vi "Simulation - Tank Level RT.vi"() -> ()   [LabVIEW 2025]
doc: "This example demonstrates a process simulation for a tank level. The process has added noise, valve deadband, lag, and deadtime. A level controller adjusts the inflow to a tank. An on/off valve serves as a drain that you can click on to operate. This s-valve represents a change in the process loading. You also can switch this VI from automatic control to manual control."
uses:
  <vilib>/addons/control/pid/pid.llb/PID Advanced (DBL).vi
  <vilib>/addons/control/pid/NI_PID_pid.lvlib
panel:
  in  "stop":bool
  in  "Tab Control":enum32{"Introduction", "Operation"}(tab)=enum."Operation"
  out "Flow sensor":bool
  in  "HV-101":bool
  out "tank level":dbl(slide)=34.9807513469828 scale=0.0..100.0 scale format="%#.2g"
  out "Valve":bool=TRUE
  in  "LCV-101":dbl(knob)=47.725128287407514 scale=0.0..100.0
  in  "Auto":bool=TRUE
  out "Process Chart":T1(graph)={"initial PV"=34.9807513469828, "SP(%)"=35.294117647058826, "output"=47.725128287407514}
  in  "Setpoint":dbl(slide)=35.294117647058826 scale=0.0..100.0
  in  "PID parameters (LIC 101)":T2={"Kc"=4.0, "Ti (min)"=0.005, "Td (min)"=0.0} {"Td (min)" format="%#.6f"; "Ti (min)" format="%#.4f"; "Kc" format="%#.4f"}
  # "Tank Level Control"
  # "Overview: This example demonstrates a process simulation for a tank level.  The process has added noise, valve deadband, lag, and deadtime.  A level controller adjusts the inflow to a tank.  An on/off valve serves as a drain that you can click on to operate.  This s-valve represents a change in the process loading.  You also can switch this VI from automatic control to manual control.\nInstructions:\n1. Run the VI.\n2. Verify the PID controller in closed-loop to track the setpoint.\n3. Change the setpoint to another value and verify the controller tracking the new setpoint.\n4. Apply a disturbance to the system by switching the valve HV 102 (click on the valve symbol). You will see the controller recovering fro the change.\n5. Change PID gains and see if you can improve its performance without going unstable.\n6. Switch to manual mode and see if you can control the level by changing the Valve LVC 101.\n7. Click Stop to stop the VI."
  # "ISA Symbology: The diagram uses the ISA Symbology used for control"
  # "Loop 101"
  # "Level Controller at the control room"
  # "Level Transmitter on the field"
  # "Level Control Valve on the field"
  # "Hand Control Valve on the field"
  # "HV"
  # "102"
  # "LCV"
  # "101"
  # "LIC"
  # "101"
  # "LT"
  # "101"
  # "Slow Leak"
  # "Click to operate"
  # "HV"
  # "102"
  # "LCV"
  # "101"
  # "LIC"
  # "101"
  # "LT"
  # "101"
  # "Manual"
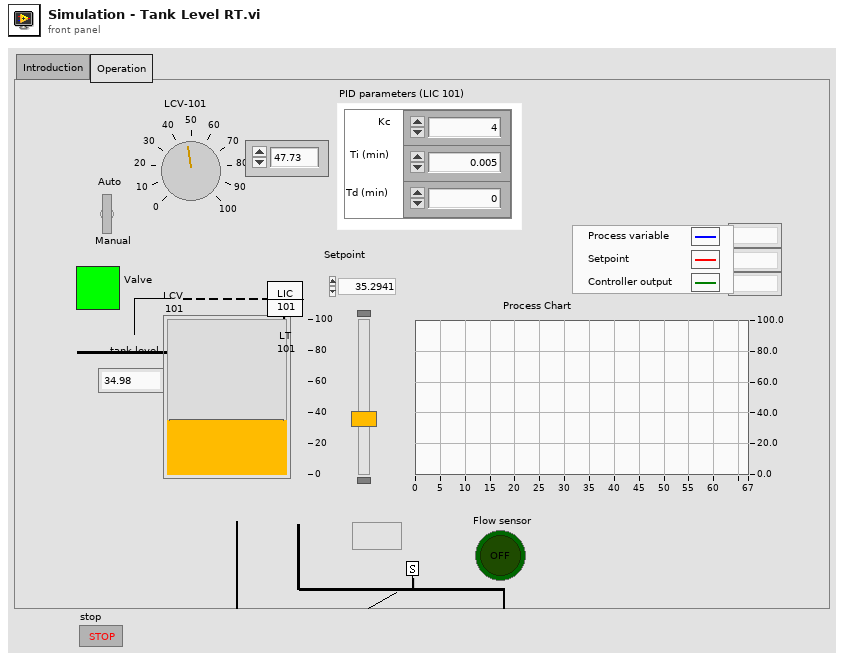
[diagram p1: front panel]
types:
  T1 = cluster{"initial PV":dbl, "SP(%)":dbl, "output":dbl}
  T2 = cluster{"Kc":dbl, "Ti (min)":dbl, "Td (min)":dbl}
  T3 = cluster{"static gain":dbl, "lag (s)":dbl, "deadtime (s)":dbl, "load":dbl, "deadband":dbl, "sensor noise":dbl, "initial PV":dbl, "plant noise":dbl}
  T4 = cluster{"Plant Output":dbl, "Setpoint":dbl, "output":dbl}
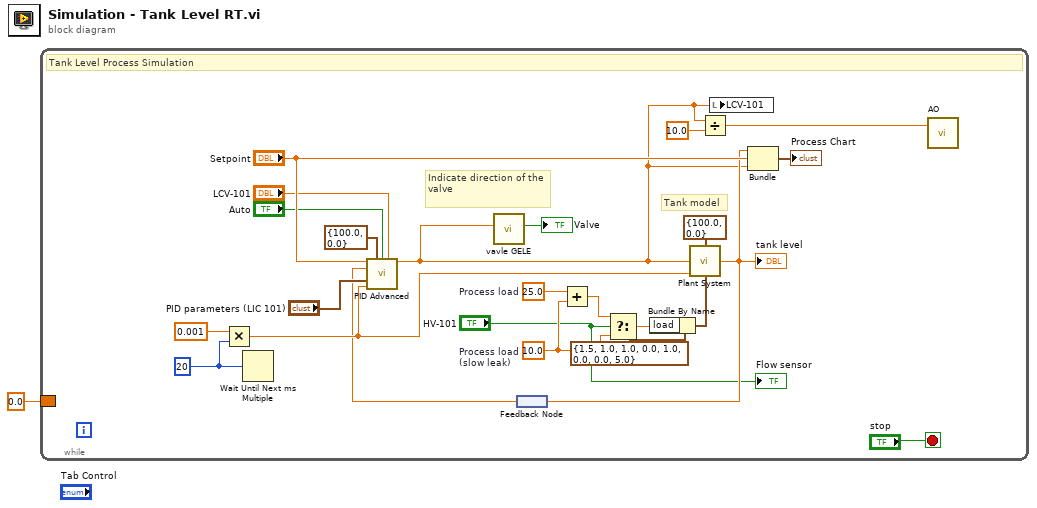
[diagram p0: block diagram]
diagram:
  n1 = while {
    border: 0.0 ("Plant Output") -> [_]
    stop <- "stop" stop-if-true
    w14 = u32 20
    w10 = 25.0  # Process load
    w11 = 10.0  # Process load (slow leak)
    # "Tank model"
    # "Indicate direction of the valve"
    # "Tank Level Process Simulation"
    n2 = Multiply(x=0.001, y=w14) -> (x*y=w13:dbl)
    n3 = Wait Until Next ms Multiple(millisecond multiple=w14) -> ()  [unwired: 1 out]
    n4 = feedback #1() -> (w5:dbl)
    n5 = call-poly <vilib>:"PID Advanced.vi"("setpoint"="Setpoint", "output range"=cluster{"output high":dbl, "output low":dbl} {"output high"=100.0, "output low"=0.0}, "auto? (T)"="Auto", "manual control"="LCV-101", "process variable"=w5, "PID gains"="PID parameters (LIC 101)", "dt (s)"=w13) -> ("output"=w3:dbl)  [unwired: 7 in, 1 out]
    n6 = call "vavle GELE.vi"("output"=w3) -> ("T=Opening"=→"Valve":bool)  [unwired: 10 in]
    n7 = Add(x=w10, y=w11) -> (x+y=w9:dbl)
    n8 = Select(t=w9, s="HV-101", f=w11) -> (s? t:f=w17:dbl)
    n9 = Bundle By Name(cluster=T3 {"static gain"=1.5, "lag (s)"=1.0, "deadtime (s)"=1.0, "load"=0.0, "deadband"=1.0, "sensor noise"=0.0, "initial PV"=0.0, "plant noise"=5.0} ("process parameters"), "load"=w17) -> (w16:T3)
    n10 = call "Plant System.vi"("output saturation range"=cluster{"output high":dbl, "output low":dbl} {"output high"=100.0, "output low"=0.0}, "Plant Input"=w3, "dt (s)"=w13, "process parameters"=w16) -> ("Plant Output"=w12:dbl)  [unwired: 11 in]
    "tank level" <- w12
    n11 = feedback-in #1(w12) -> ()
    n12 = Divide(x=w3, y=10.0) -> (x/y=w6:dbl)
    n13 = local write "LCV-101"(w3) -> ()
    n14 = Bundle("Plant Output"=w12, "Setpoint"="Setpoint", "output"=w3) -> (→"Process Chart":T4)  [unwired: 1 in]
    n15 = call "AO"("data"=w6) -> ()  [unwired: 17 in, 2 out]
    "Flow sensor" <- "HV-101"
  }
